vi "Get_cage_size_text_from_Geometry_data.vi"(2 "Error In":errorcluster, 3 "Geometry":T1 {"Cage type" items=["Round", "Square", "Donut-maze", "T-maze", "Sociability maze", ""]}) -> (0 "Error Out":errorcluster, 1 "Cage size text":string)   [LabVIEW 2018, in "Tracker.lvlib"]
uses:
  Tracker.lvlib
  Controls/CTL_Segmented_plot_parameters_2.ctl
  Libraries/Cage Diagram/Typedefs/CTL_Cage_type.ctl
  Controls/CTL_Cage_all_segmentation_params_set.ctl
  Controls/CTL_Segmented_plot_parameters_2_(round_d1).ctl
  Common_Resources.lvlib
  Libraries/Cage Diagram/Cage Diagram.lvlib
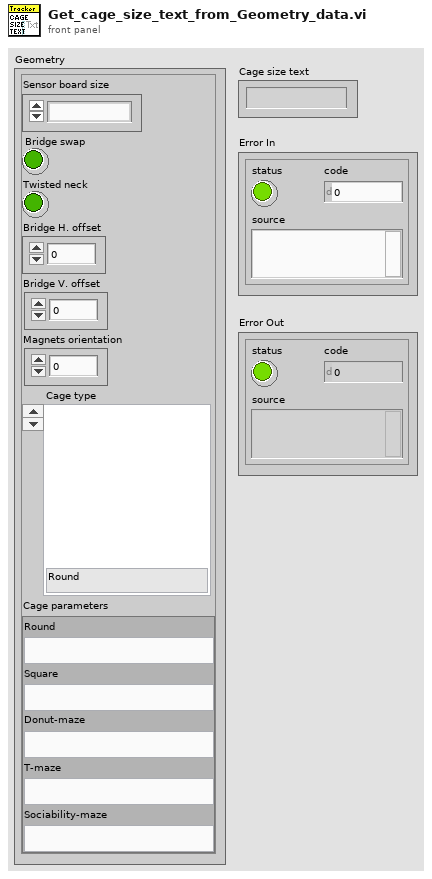
[diagram p1: front panel]
types:
  T1 = typedef "Common_Resources.lvlib/CTL_Segmented_plot_parameters_2.ctl" = cluster{"Sensor board size":enum16{"", "Large"}, "Bridge swap":bool, "Twisted neck":bool, "Bridge H. offset":sgl, "Bridge V. offset":sgl, "Magnets orientation":sgl, "Cage type":T2, "Cage parameters":T3}
  T2 = typedef "Cage Diagram.lvlib/CTL_Cage_type.ctl" = u16
  T3 = typedef "Common_Resources.lvlib/CTL_Cage_all_segmentation_params_set.ctl" = cluster{"Round":variant, "Square":variant, "Donut-maze":variant, "T-maze":variant, "Sociability-maze":variant}
  T4 = typedef "Common_Resources.lvlib/CTL_Segmented_plot_parameters_2_(round_d1).ctl" = cluster{"Cage diameter, mm":u16, "Starting angle BORDER":i16, "Starting angle MIDFIELD":i16, "Radius, mm MIDFIELD":u16, "Radius, mm CENTER":u16, "N segments BORDER":u8, "N segments MIDFIELD":u8, "R-gap, mm":sgl}
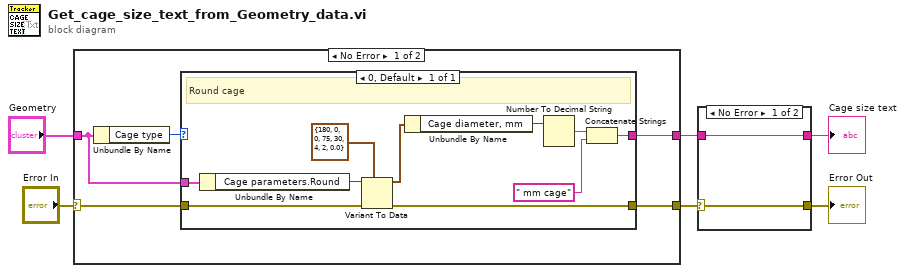
[diagram p0: block diagram]
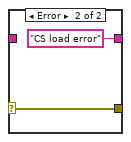
[diagram p2: hidden frame]
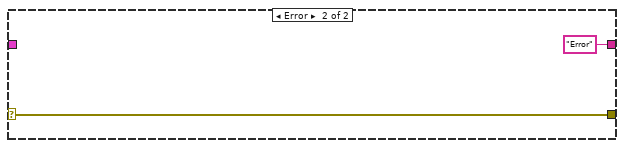
[diagram p3: hidden frame]
diagram:
  n1 = case shown="No Error" "Error In" {
    selector: "Error In" -> [w9 w23]
    tunnel: "Geometry" -> [w10 _]
    tunnel: [w8 "Error"] -> w3
    tunnel: [w7 w23] -> w4
    frame No Error {
      n2 = Unbundle By Name(w10) -> ("Cage type"=w11:T2)
      n3 = case shown="0, Default" w11 {
        tunnel: w10 -> [w21]
        tunnel: w9 -> [w18]
        tunnel: [w13] -> w8
        tunnel: [w12] -> w7
        frame 0, Default {
          # "Round cage"
          n4 = Unbundle By Name(w21) -> ("Cage parameters.Round"=w19:variant)
          n5 = Variant To Data(error in=w18, type=T4 {"Cage diameter, mm"=180, "Starting angle BORDER"=0, "Starting angle MIDFIELD"=0, "Radius, mm MIDFIELD"=75, "Radius, mm CENTER"=30, "N segments BORDER"=4, "N segments MIDFIELD"=2, "R-gap, mm"=0.0} ("Radial segmentation parameters"), Variant=w19) -> (data=w17:T4, error out=w12:errorcluster)
          n6 = Unbundle By Name(w17) -> ("Cage diameter, mm"=w16:u16)
          n7 = Number To Decimal String(number=w16) -> (decimal integer string=w15:string)  [unwired: 1 in]
          n8 = Concatenate Strings(w15, " mm cage" ("string")) -> (w13:string)
        }
      }
    }
    frame Error {
    }
  }
  n9 = case shown="No Error" w4 {
    selector: w4 -> [w25 w27]
    tunnel: w3 -> [w24 _]
    tunnel: [w25 w27] -> w2
    tunnel: [w24 "CS load error"] -> w1
    frame No Error {
    }
    frame Error {
    }
  }
  "Error Out" <- w2
  "Cage size text" <- w1
